vi "4431 Calculate buffer info.vi"(9 "sample mode":i32, 10 "sampling info":cluster{"Fs":dbl, "#s":dbl}, 11 "AI Buffer Size (S)":i32) -> (1 "Fs":dbl, 2 "Numeric 2":dbl, 3 "Numeric 3":dbl, 4 "Numeric":dbl, 5 "Boolean":bool)   [LabVIEW 2016]
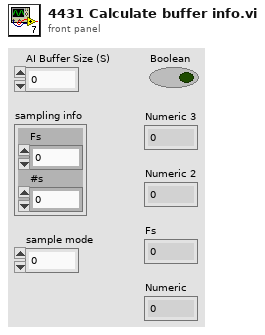
[diagram p1: front panel]
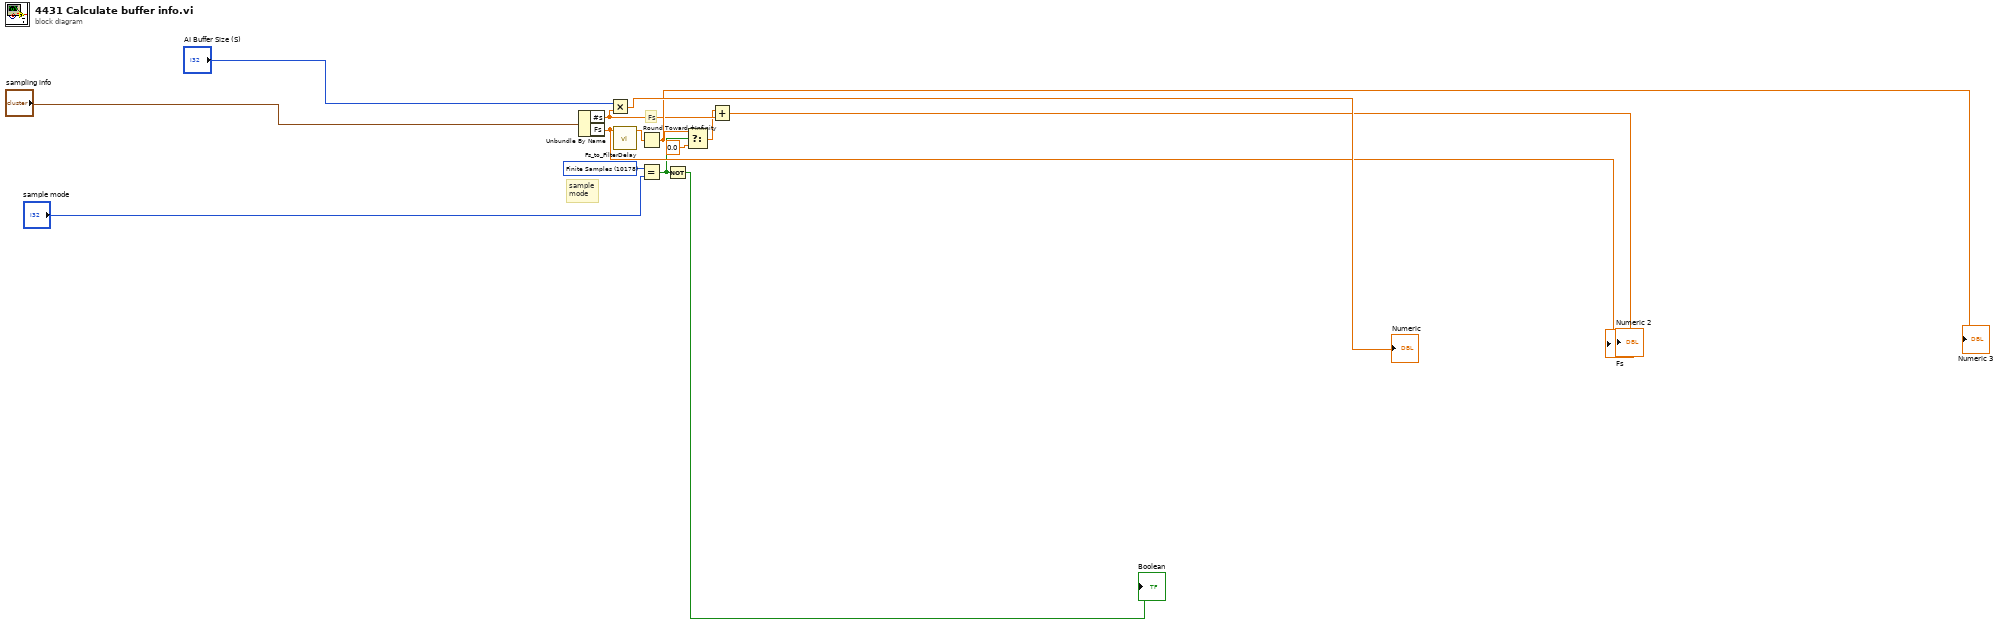
[diagram p0: block diagram]
diagram:
  w4 = 10178 items=["Finite Samples"=10178, "Continuous Samples"=10123] ("sample mode 2")
  # "Fs"
  # "sample\nmode"
  n1 = Unbundle By Name("sampling info") -> ("#s"=w7:dbl, "Fs"=w12:dbl)
  "Fs" <- w12
  n2 = Multiply(x="AI Buffer Size (S)", y=w7) -> (x*y=→"Numeric":dbl)
  n3 = call "Fs_to_FilterDelay.vi"("Fs"=w12) -> ("Total Filter Delay (samples)"=w1:dbl)  [unwired: 10 in]
  n4 = Round Toward +Infinity(x=w1) -> (ceil(x): smallest int >= x=w10:dbl)
  "Numeric 3" <- w10
  n5 = Equal?(x=w4, y="sample mode") -> (x = y?=w8:bool)
  n6 = Not(x=w8) -> (.not. x?=→"Boolean":bool)
  n7 = Select(t=w10, s=w8, f=0.0) -> (s? t:f=w3:dbl)
  n8 = Add(x=w3, y=w7) -> (x+y=→"Numeric 2":dbl)
